vi "WPILogGetStartControl.vi"(8 "error in (no error)":errorcluster, 11 "raw data":u8[](array[numeric])) -> (0 "error out":errorcluster, 2 "remaining bytes":u8[](array[numeric]), 3 "Control Entry":T1)   [LabVIEW 2020]
uses:
  Typedef/Control Header.ctl
panel:
  out "Type":u8
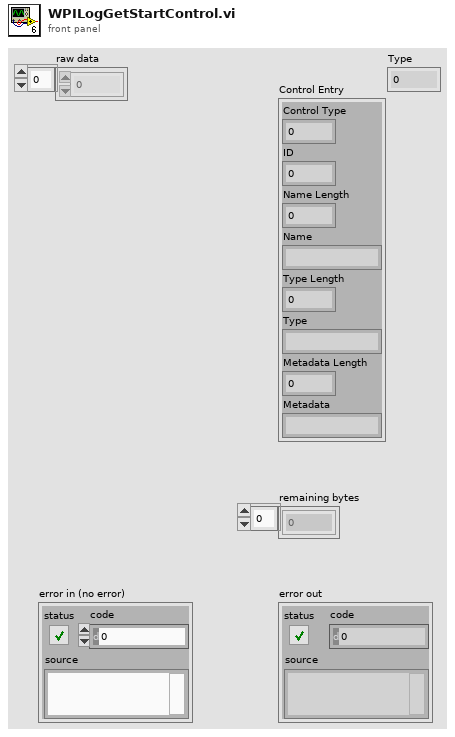
[diagram p1: front panel]
types:
  T1 = typedef "Control Header.ctl" = cluster{"Control Type":u8, "ID":u32, "Name Length":u32, "Name":string, "Type Length":u32, "Type":string, "Metadata Length":u32, "Metadata":string}
  T2 = enum16{"big-endian, network order", "native, host order", "little-endian"}
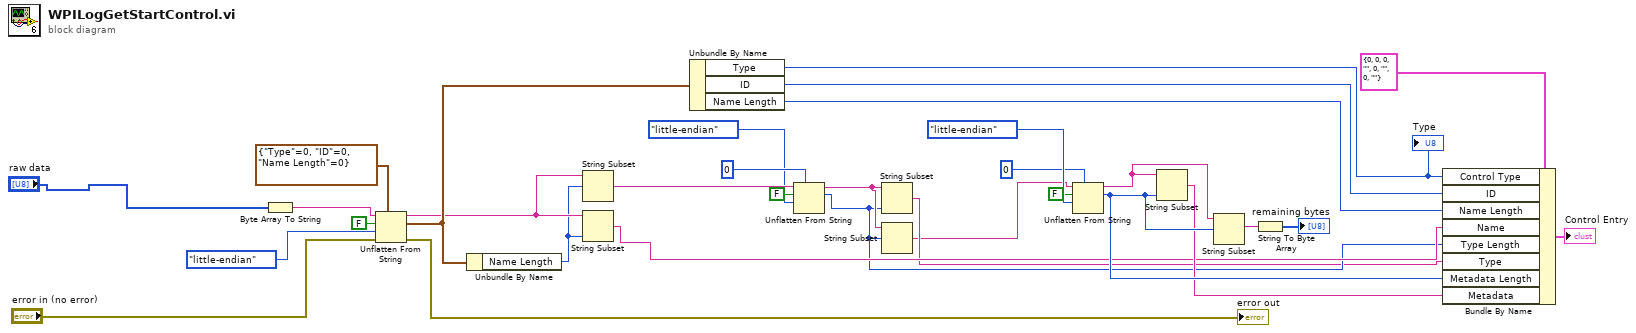
[diagram p0: block diagram]
diagram:
  n1 = Byte Array To String(unsigned byte array="raw data") -> (string=w9:string)
  n2 = Unflatten From String(type=cluster{"Type":u8, "ID":u32, "Name Length":u32} {"Type"=0, "ID"=0, "Name Length"=0}, binary string=w9, data includes array or string size? (T)=FALSE, byte order (0:big-endian, network order)=T2."little-endian", error in (no error)="error in (no error)") -> (rest of the binary string=w13:string, value=w21:cluster{"Type":u8, "ID":u32, "Name Length":u32}, error out=→"error out":errorcluster)
  n3 = Unbundle By Name(w21) -> ("Name Length"=w12:u32)
  n4 = String Subset(string=w13, offset (0)=w12) -> (substring=w15:string)  [unwired: 1 in]
  n5 = String Subset(string=w13, length (rest)=w12) -> (substring=w20:string)  [unwired: 1 in]
  n6 = Unbundle By Name(w21) -> ("Type"=w22:u8, "ID"=w23:u32, "Name Length"=w24:u32)
  "Type" <- w22
  n7 = Unflatten From String(type=u32 0, binary string=w15, data includes array or string size? (T)=FALSE, byte order (0:big-endian, network order)=T2."little-endian") -> (rest of the binary string=w18:string, value=w3:u32)  [unwired: 1 in, 1 out]
  n8 = String Subset(string=w18, length (rest)=w3) -> (substring=w2:string)  [unwired: 1 in]
  n9 = String Subset(string=w18, offset (0)=w3) -> (substring=w1:string)  [unwired: 1 in]
  n10 = Unflatten From String(type=u32 0, binary string=w1, data includes array or string size? (T)=FALSE, byte order (0:big-endian, network order)=T2."little-endian") -> (rest of the binary string=w4:string, value=w29:u32)  [unwired: 1 in, 1 out]
  n11 = String Subset(string=w4, length (rest)=w29) -> (substring=w28:string)  [unwired: 1 in]
  n12 = String Subset(string=w4, offset (0)=w29) -> (substring=w30:string)  [unwired: 1 in]
  n13 = String To Byte Array(string=w30) -> (unsigned byte array=→"remaining bytes":u8[])
  n14 = Bundle By Name(cluster=T1 {"Control Type"=0, "ID"=0, "Name Length"=0, "Name"="", "Type Length"=0, "Type"="", "Metadata Length"=0, "Metadata"=""}, "Control Type"=w22, "ID"=w23, "Name Length"=w24, "Name"=w20, "Type Length"=w3, "Type"=w2, "Metadata Length"=w29, "Metadata"=w28) -> (→"Control Entry":T1)
